vi "GEN_2D_Histo_Bins.vi"(3 "Error In":errorcluster, 5 "Bins parameters":T1={"Xmax"=110.0, "Xmin"=-110.0, "Ymax"=110.0, "Ymin"=-110.0, "# bins per axis"=11}) -> (0 "Error Out":errorcluster, 1 "Y bins (center)":dbl[](array[numeric]), 2 "X bins (center)":dbl[](array[numeric]))   [LabVIEW 2018, in "Tracker.lvlib"]
uses:
  Tracker.lvlib
  Controls/CTL_2D_bins_parameters.ctl
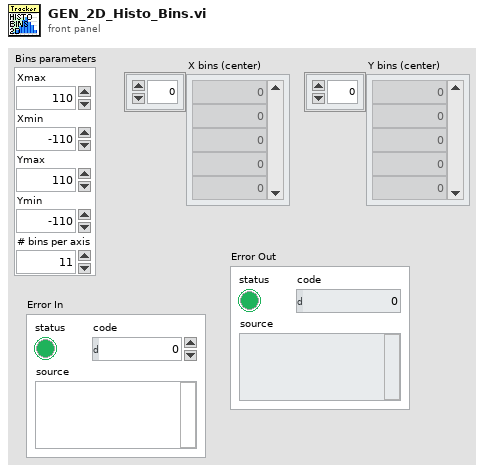
[diagram p1: front panel]
types:
  T1 = typedef "Tracker.lvlib/CTL_2D_bins_parameters.ctl" = cluster{"Xmax":dbl, "Xmin":dbl, "Ymax":dbl, "Ymin":dbl, "# bins per axis":i32}
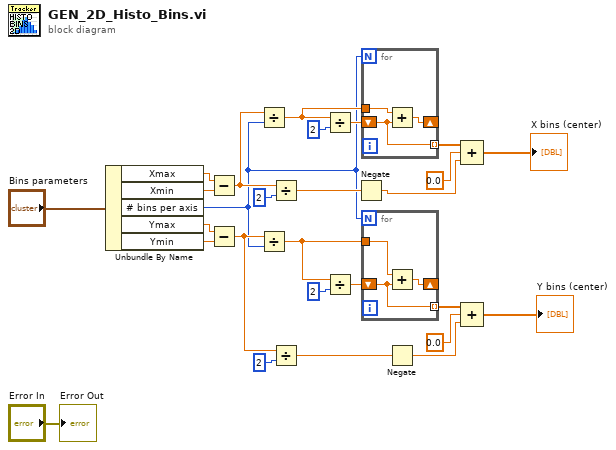
[diagram p0: block diagram]
diagram:
  n1 = Unbundle By Name("Bins parameters") -> ("Xmax"=w21:dbl, "Xmin"=w20:dbl, "# bins per axis"=w2:i32, "Ymax"=w4:dbl, "Ymin"=w3:dbl)
  n2 = Subtract(x=w21, y=w20) -> (x-y=w17:dbl)
  n3 = Subtract(x=w4, y=w3) -> (x-y=w10:dbl)
  n4 = Divide(x=w17, y=w2) -> (x/y=w25:dbl)
  n5 = Divide(x=w10, y=w2) -> (x/y=w7:dbl)
  n6 = Divide(x=w17, y=2) -> (x/y=w16:dbl)
  n7 = Divide(x=w10, y=2) -> (x/y=w11:dbl)
  n8 = Divide(x=w25, y=2) -> (x/y=w27:dbl)
  n9 = Divide(x=w7, y=2) -> (x/y=w5:dbl)
  n10 = Negate(x=w16) -> (-x=w15:dbl)
  n11 = for {
    N: w2 -> [_]
    tunnel: w25 -> [w30]
    tunnel: [w28] -> w26 mode=indexing
    shift-right: [w29] -> _
    shift-left: w27 -> [w28]
    n12 = Add(x=w30, y=w28) -> (x+y=w29:dbl)
  }
  n13 = for {
    N: w2 -> [_]
    tunnel: w7 -> [w33]
    tunnel: [w31] -> w6 mode=indexing
    shift-right: [w32] -> _
    shift-left: w5 -> [w31]
    n14 = Add(x=w33, y=w31) -> (x+y=w32:dbl)
  }
  n15 = Negate(x=w11) -> (-x=w12:dbl)
  n16 = Compound Arithmetic op=ADD(w26, 0.0, w15) -> (→"X bins (center)":dbl[])
  n17 = Compound Arithmetic op=ADD(w6, 0.0, w12) -> (→"Y bins (center)":dbl[])
  "Error Out" <- "Error In"
